vi "gfitsio-resize-image.vi"(4 "image data type":T1 items=["<invalid type>"=0, "BYTE_IMG  (U8)"=8, "SHORT_IMG  (I16)"=16, "USHORT_IMG  (U16)"=20, "LONG_IMG  (I32)"=32, "ULONG_IMG  (U32)"=40, "FLOAT_IMG  (SGL)"=-32, "DOUBLE_IMG  (DBL)"=-64], 6 "naxes":i32[](array[numeric]), 8 "error in (no error)":errorcluster, 11 "gfits refnum":T2) -> (0 "error out":errorcluster, 3 "dup gfits refnum":T2)   [LabVIEW 2013, in "gfitsio.lvlib"]
doc: "Modify the size, dimensions, and/or data type of the current primary array or image extension. If the new image, as specified by the input arguments, is larger than the current existing image in the FITS file then zero fill data will be inserted at the end of the current image and any following extensions will be moved further back in the file. Similarly, if the new image is smaller than the current image then any following extensions will be shifted up towards the beginning of the FITS file and the image data will be truncated to the new size. This routine rewrites the BITPIX, NAXIS, and NAXISn keywords with the appropriate values for the new image."
uses:
  gfitsio.lvlib
  gfitsio-refnum.ctl
  cfitsio-bitpix.ctl
  gfitsio-error-codes.ctl
  gfitsio.dll
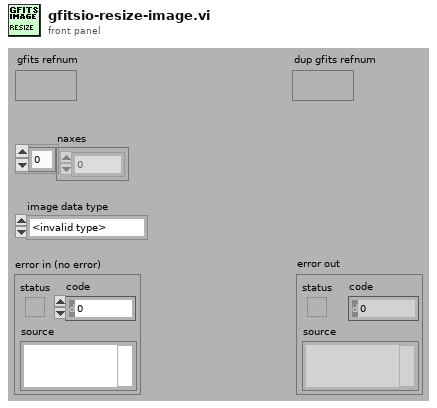
[diagram p1: front panel]
types:
  T1 = typedef "gfitsio.lvlib/cfitsio-bitpix.ctl" = i32
  T2 = typedef "gfitsio.lvlib/gfitsio-refnum.ctl" = refnum<k1>
  T3 = typedef "gfitsio.lvlib/gfitsio-error-codes.ctl" = i32
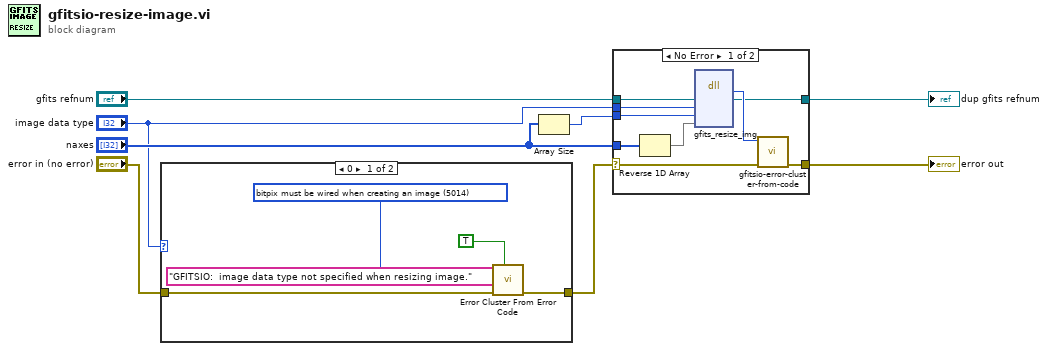
[diagram p0: block diagram]
diagram:
  n1 = case shown="0" "image data type" {
    tunnel: "error in (no error)" -> [w12 w14]
    tunnel: [w13 w14] -> w4
    frame 0 {
      w11 = T3 5014 items=["no error"=0, "dimensionality conflict"=5001, "fpixel out of image bounds"=5002, "lpixel out of image bounds"=5003, "increment size larger than image"=5004, "increment must be greater than zero"=5005, "fpixel must specify lower left corner"=5006, "named HDU not found"=5007, "specified row is past the end of the table"=5008, "wrong number of elements for column"=5009, "column is not scalar"=5010, "duplicate HDU name"=5011, "invalid table type"=5012, "row counting starts at 1"=5013, "bitpix must be wired when creating an image"=5014] ("Ring")
      n2 = call <vilib>:"Error Cluster From Error Code.vi"("show call chain? (False)"=TRUE, "error in (no error)"=w12, "error message (\"\")"="GFITSIO:  image data type not specified when resizing image." ("error message (\"\")"), "error code (0)"=w11) -> ("error out"=w13:errorcluster)  [unwired: 5 out]
    }
    frame Default {
    }
  }
  n3 = Array Size(array="naxes") -> (size(s)=w6:i32)
  n4 = case shown="No Error" w4 {
    selector: w4 -> [w21 w25]
    tunnel: [w23 w25] -> w2
    tunnel: "naxes" -> [w17 _]
    tunnel: "gfits refnum" -> [w19 w24]
    tunnel: [w20 w24] -> w1
    tunnel: w6 -> [w18 _]
    tunnel: "image data type" -> [w16 _]
    frame No Error {
      n5 = Reverse 1D Array(array=w17) -> (reversed array=w15:i32[])
      n6 = dll-call lib="H:/Shared Code/LabVIEW GFITSIO/gfitsio.dll" fn="gfits_resize_img"("refnum"=w19, "bitpix"=w16, "naxis"=w18, "naxes"=w15) -> ("return type"=w22:i32, "refnum"=w20:T2)  [unwired: 5 in, 3 out]
      n7 = call "gfitsio-error-cluster-from-code.vi"("error in (no error)"=w21, "error code"=w22) -> ("error out"=w23:errorcluster)  [unwired: 9 out]
    }
    frame Error {
    }
  }
  "error out" <- w2
  "dup gfits refnum" <- w1
